vi "TxtLog.vi"() -> ()   [LabVIEW 2020]
uses:
  <vilib>/Utility/error.llb/DialogType.ctl
panel:
  out "error out":errorcluster
  in  "error in":errorcluster
  in  "LogFile":path
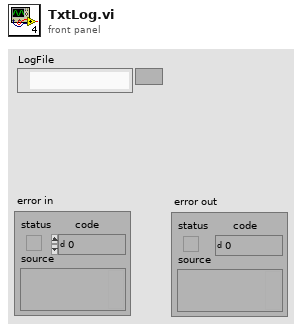
[diagram p1: front panel]
types:
  T1 = typedef "DialogType.ctl" = u16
  T2 = enum16{"open", "replace", "create", "open or create", "replace or create", "replace or create with confirmation"}
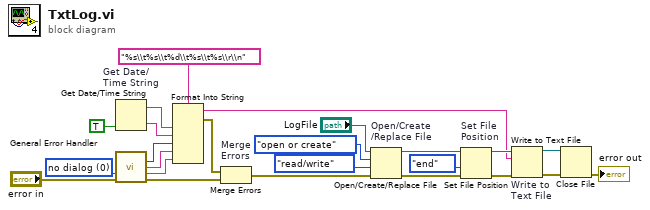
[diagram p0: block diagram]
diagram:
  w12 = T1 0 items=["no dialog", "OK message", "continue or stop message", "OK message + warnings", "continue/stop + warnings"] ("type of dialog (OK msg:1)")
  n1 = Get Date/Time String "Get Date/\nTime String"(want seconds? (F)=TRUE ("want seconds?")) -> (date string=w10:string, time string=w9:string)  [unwired: 2 out]
  n2 = call <vilib>:"General Error Handler.vi"("type of dialog (OK msg:1)"=w12, "error in (no error)"="error in") -> ("code out"=w7:i32, "source out"=w6:string, "message"=w5:string, "error out"=w2:errorcluster)  [unwired: 9 in, 1 out]
  n3 = Format Into String(format string="%s\\t%s\\t%d\\t%s\\t%s\\r\\n", w10, w9, w7, w6, w5) -> (resulting string=w4:string, error out=w3:errorcluster)  [unwired: 2 in]
  n4 = Merge Errors "Merge\nErrors"(w3, w2) -> (w1:errorcluster)
  n5 = Open/Create/Replace File "Open/Create\n/Replace File"(file path (use dialog)="LogFile", error in=w1, operation (0:open)=T2."open or create", access (0:read/write)=enum16{"read/write", "read-only", "write-only"}."read/write") -> (refnum out=w19:refnum<file>, error out=w18:errorcluster)  [unwired: 3 out]
  n6 = Set File Position "Set File\nPosition"(refnum=w19, from (0:start)=enum16{"start", "end", "current"}."end", error in=w18) -> (refnum out=w16:refnum<file>, error out=w15:errorcluster)  [unwired: 1 out]
  n7 = Write to Text File "Write to \nText File"(file (use dialog)=w16, text=w4, error in=w15) -> (refnum out=w21:refnum<file>, error out=w20:errorcluster)  [unwired: 2 out]
  n8 = Close File(refnum=w21, error in=w20) -> (error out=→"error out":errorcluster)  [unwired: 1 out]
